vi "Scope_1SDI_v00.vi"(0 "Scope+Safety":T1={"Safety First"={"lim reset"=FALSE, "no limit"=FALSE, "pos slew rate * dt"=12, "neg slew rate * dt"=-12, "Count(Ticks)"=0}, "Scope IPs"={"Trigger Direction"=enum."minus-plus", "Trigger Delay (ms)"=0.0, "Aquisition Rate (kHz)"=4000.0, "Trigger Offset (V)"=0.0, "Scale Offset"={"Scaling"={"Error signal"=1, "Output"=0, "DC Monitor"=1, "Threshold"=1}, "Offset"={"Error Signal"=0, "Output"=0, "DC Monitor"=0, "Threshold"=0}}}}, 9 "Scope":T2, 11 "Lock Select":T4, 13 "XY HD ON":bool, 14 "1SDI Data":u64[](array[numeric])) -> (1 "xy HD A":cluster{i16[], i16[]}(graph), 2 "xy HD B":cluster{i16[], i16[]}(graph), 3 "Scope OP 1SDI":cluster{dbl[], dbl[]}[](graph), 6 "Scope 1SDI ON":bool, 8 "error":dbl[](array[numeric]), 15 "Scope 1SDI FPGA":T3)   [LabVIEW 2013]
doc: "Creates an oscilliscope graph from the FIFO data, as well as packages data structures for FPGA_Cavities via the reference."
uses:
  Strict Type Defs/Lock Select 1SDI.ctl
  Strict Type Defs/Lock or Hold.ctl
  Strict Type Defs/Scope and Safety.ctl
panel:
  out "Scope OPs (for saving)":cluster{dbl[], i16[], i16[], i16[], i16[]}
  in  "Scope":T3={"Trigger Direction"=enum."minus-plus", "Delay"=0, "Aquisition Rate (Ticks)"=20, "Offset"=0, "Channel"=0, "Channel Selector"={"Channel 1"=0, "Channel 2"=0, "Channel 3"=0, "Channel 4"=0}}
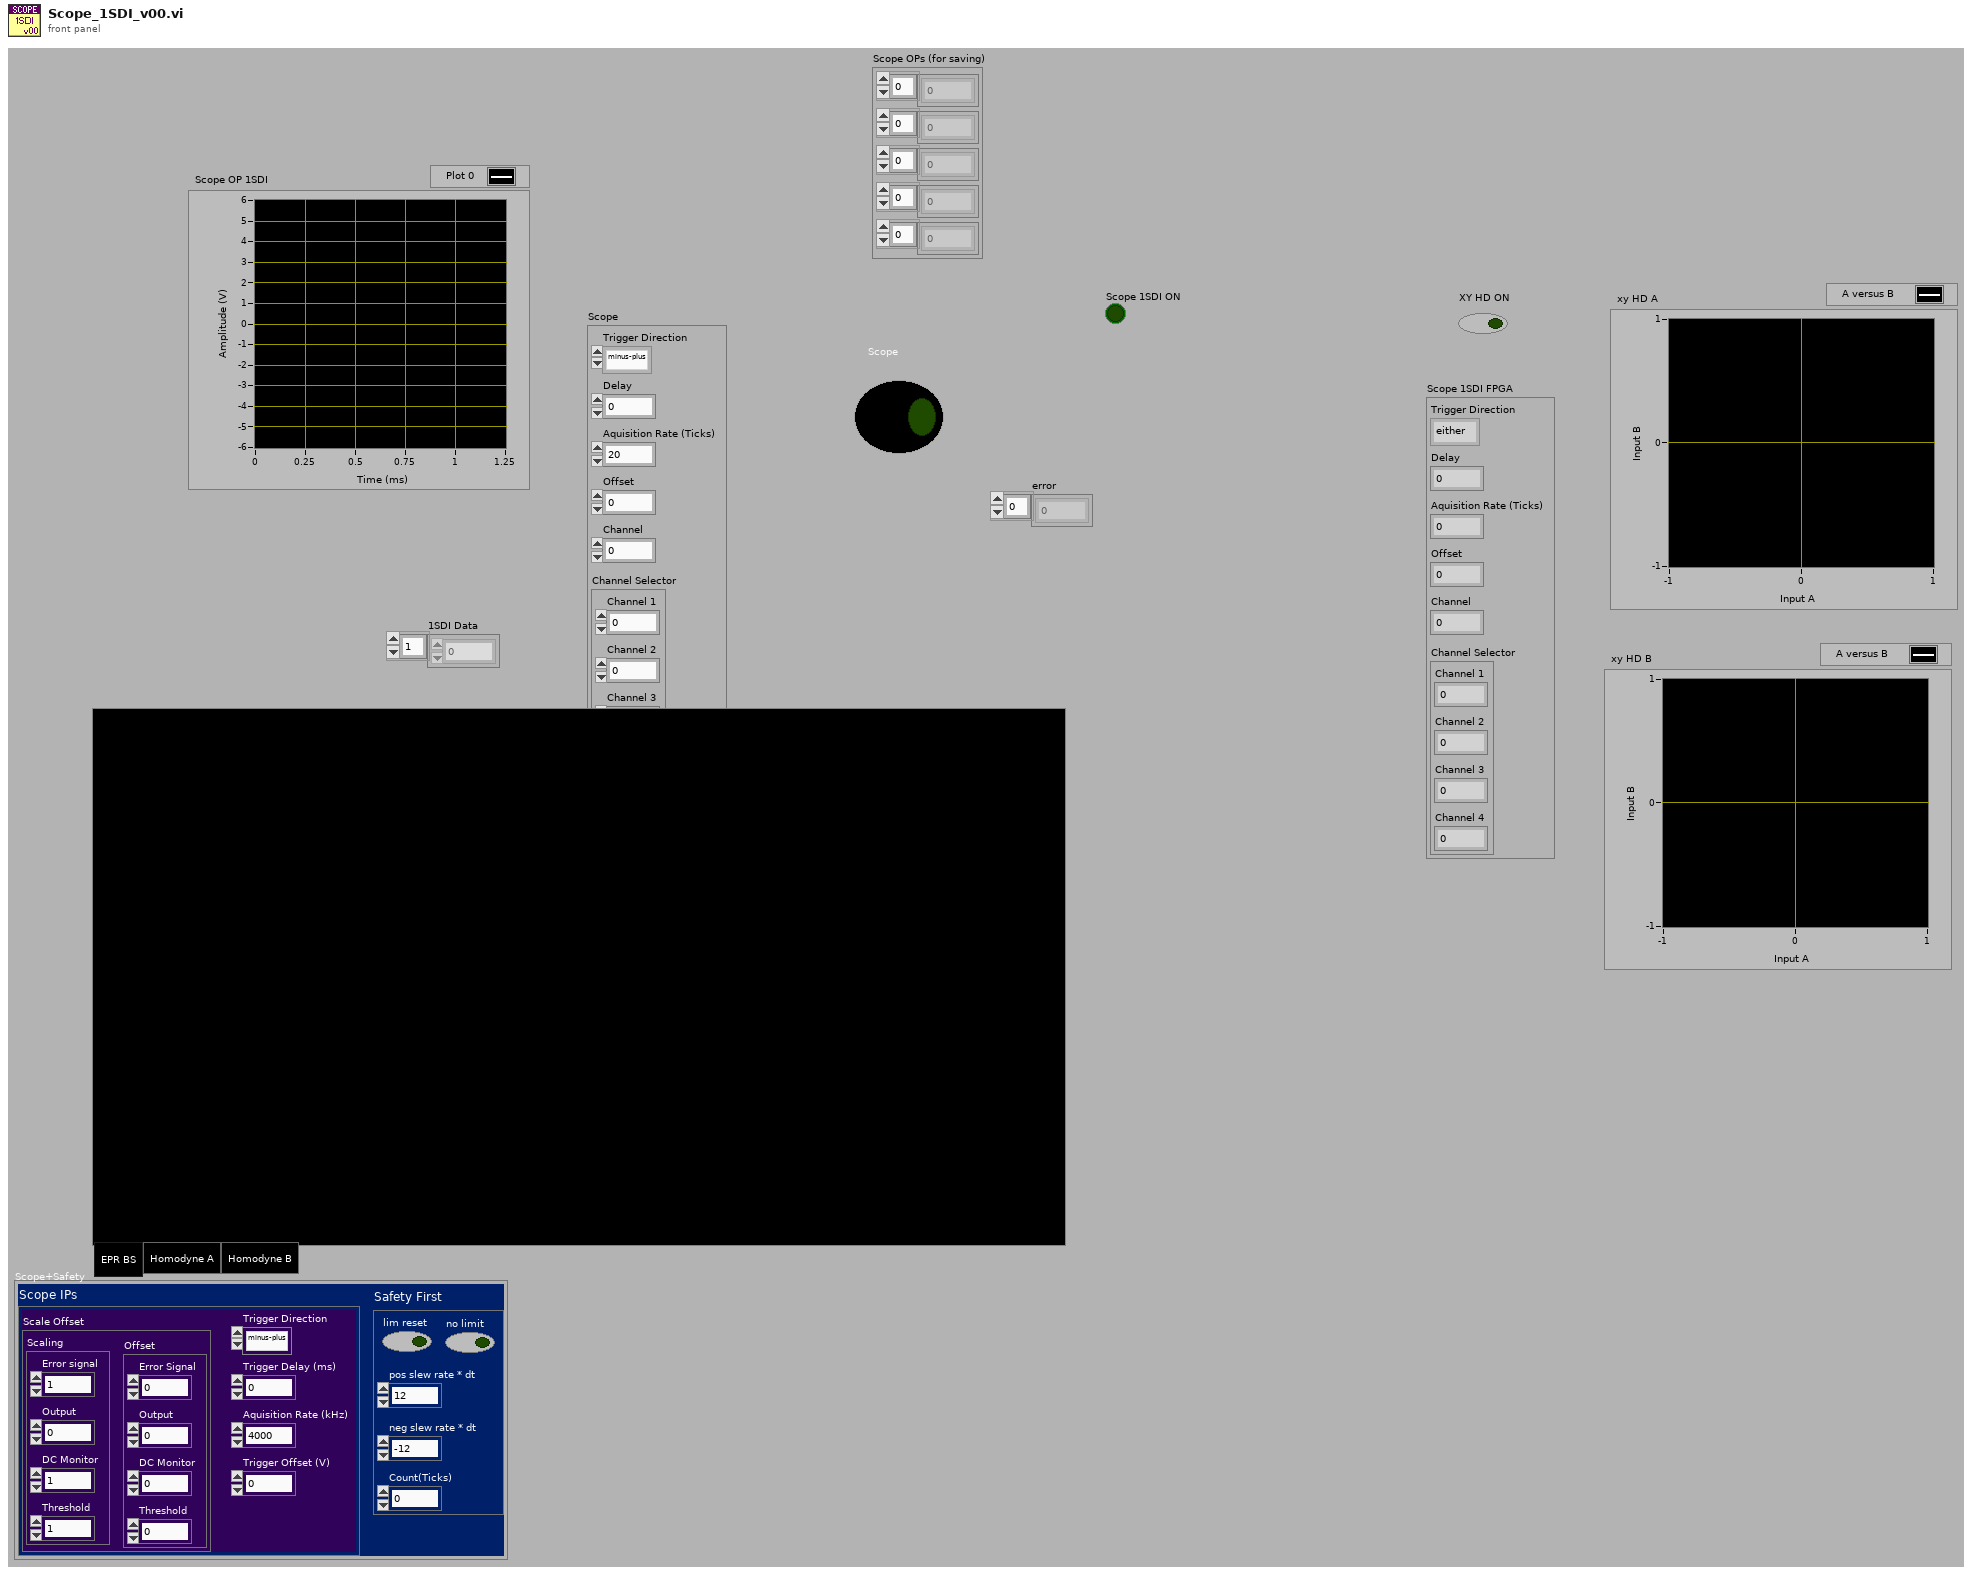
[diagram p1: front panel]
types:
  T1 = typedef "Scope and Safety.ctl" = cluster{"Safety First":cluster{"lim reset":bool, "no limit":bool, "pos slew rate * dt":i16, "neg slew rate * dt":i16, "Count(Ticks)":u32}, "Scope IPs":cluster{"Trigger Direction":enum8{"either", "minus-plus", "plus-minus"}, "Trigger Delay (ms)":dbl, "Aquisition Rate (kHz)":dbl, "Trigger Offset (V)":dbl, "Scale Offset":cluster{"Scaling":cluster{"Error signal":i16, "Output":i16, "DC Monitor":i16, "Threshold":i16}, "Offset":cluster{"Error Signal":i16, "Output":i16, "DC Monitor":i16, "Threshold":i16}}}}
  T2 = typedef "Lock or Hold.ctl" = bool
  T3 = cluster{"Trigger Direction":enum8{"either", "minus-plus", "plus-minus"}, "Delay":u32, "Aquisition Rate (Ticks)":u32, "Offset":i16, "Channel":i32, "Channel Selector":cluster{"Channel 1":i32, "Channel 2":i32, "Channel 3":i32, "Channel 4":i32}}
  T4 = typedef "Lock Select 1SDI.ctl" = enum32{"EPR BS", "Homodyne A", "Homodyne B"}
  T5 = cluster{"Channel 1":i32, "Channel 2":i32, "Channel 3":i32, "Channel 4":i32}
  T6 = cluster{"Trigger Direction":enum8{"either", "minus-plus", "plus-minus"}, "Trigger Delay (ms)":dbl, "Aquisition Rate (kHz)":dbl, "Trigger Offset (V)":dbl, "Scale Offset":cluster{"Scaling":cluster{"Error signal":i16, "Output":i16, "DC Monitor":i16, "Threshold":i16}, "Offset":cluster{"Error Signal":i16, "Output":i16, "DC Monitor":i16, "Threshold":i16}}}
  T7 = cluster{"Error signal":i16, "Output":i16, "DC Monitor":i16, "Threshold":i16}
  T8 = cluster{"Error Signal":i16, "Output":i16, "DC Monitor":i16, "Threshold":i16}
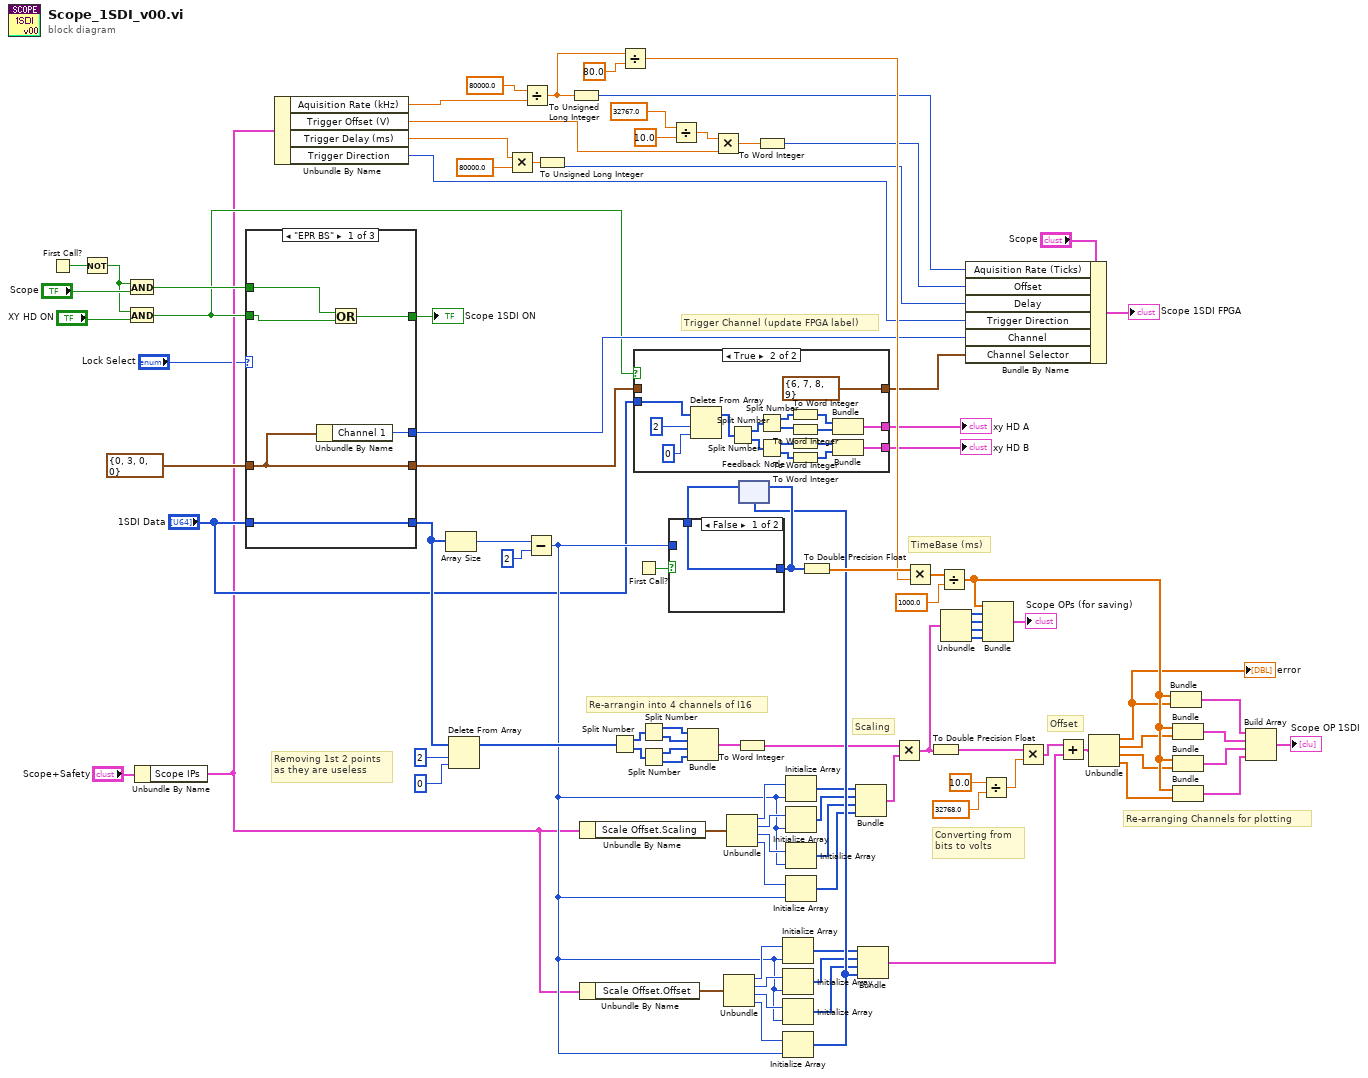
[diagram p0: block diagram]
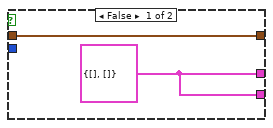
[diagram p2: hidden frame]
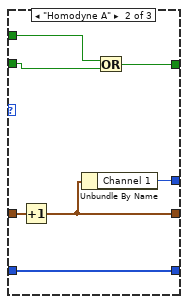
[diagram p4: hidden frame]
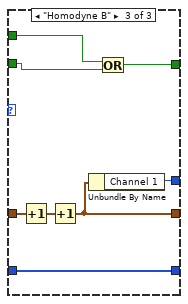
[diagram p5: hidden frame]
diagram:
  # "Trigger Channel (update FPGA label)"
  # "TimeBase (ms)"
  # "Re-arranging Channels for plotting"
  # "Re-arrangin into 4 channels of I16"
  # "Converting from\nbits to volts"
  # "Offset"
  # "Scaling"
  # "Removing 1st 2 points\nas they are useless"
  n1 = First Call?() -> (First Call?: T/F=w17:bool)
  n2 = Not(x=w17) -> (.not. x?=w11:bool)
  n3 = And(x=w11, y="Scope") -> (x .and. y?=w16:T2)
  n4 = And(x=w11, y="XY HD ON") -> (x .and. y?=w8:bool)
  n5 = Unbundle By Name("Scope+Safety") -> ("Scope IPs"=w3:T6)
  n6 = case shown="\"EPR BS\"" "Lock Select" {
    tunnel: [w105 w111 w115] -> w26
    tunnel: "1SDI Data" -> [w105 w111 w115]
    tunnel: [w100 w107 w114] -> w19
    tunnel: T5 {"Channel 1"=0, "Channel 2"=3, "Channel 3"=0, "Channel 4"=0} ("Channel Selector") -> [w101 w112 w120]
    tunnel: [w101 w106 w113] -> w10
    tunnel: w16 -> [w102 w108 w116]
    tunnel: [w104 w110 w118] -> w14
    tunnel: w8 -> [w103 w109 w117]
    frame "EPR BS" {
      n7 = Unbundle By Name(w101) -> ("Channel 1"=w100:i32)
      n8 = Or(x=w102, y=w103) -> (x .or. y?=w104:T2)
    }
    frame "Homodyne A" {
      n9 = Increment(x=w112) -> (x+1=w106:T5)
      n10 = Unbundle By Name(w106) -> ("Channel 1"=w107:i32)
      n11 = Or(x=w108, y=w109) -> (x .or. y?=w110:T2)
    }
    frame "Homodyne B" {
      n12 = Increment(x=w120) -> (x+1=w119:T5)
      n13 = Increment(x=w119) -> (x+1=w113:T5)
      n14 = Unbundle By Name(w113) -> ("Channel 1"=w114:i32)
      n15 = Or(x=w116, y=w117) -> (x .or. y?=w118:T2)
    }
  }
  "Scope 1SDI ON" <- w14
  n16 = Unbundle By Name(w3) -> ("Aquisition Rate (kHz)"=w98:dbl, "Trigger Offset (V)"=w93:dbl, "Trigger Delay (ms)"=w91:dbl, "Trigger Direction"=w20:enum8{"either", "minus-plus", "plus-minus"})
  n17 = Array Size(array=w26) -> (size(s)=w84:i32)
  n18 = Delete From Array(array=w26, length=2, index=0) -> (array with subset deleted=w30:u64[])  [unwired: 1 out]
  n19 = Multiply(x=w91, y=80000.0) -> (x*y=w92:dbl)
  n20 = Divide(x=80000.0, y=w98) -> (x/y=w88:dbl)
  n21 = Subtract(x=w84, y=2) -> (x-y=w13:i32)
  n22 = To Unsigned Long Integer(number=w92) -> (unsigned 32bit integer=w21:u32)
  n23 = To Unsigned Long Integer(number=w88) -> (unsigned 32bit integer=w23:u32)
  n24 = Unbundle By Name(w3) -> ("Scale Offset.Scaling"=w55:T7)
  n25 = Unbundle By Name(w3) -> ("Scale Offset.Offset"=w39:T8)
  n26 = Split Number(x=w30) -> (hi(x)=w32:u32[], lo(x)=w31:u32[])
  n27 = Divide(x=w88, y=80.0) -> (x/y=w29:dbl)
  n28 = case shown="True" w8 {
    tunnel: w10 -> [w122 _]
    tunnel: [w122 T5 {"Channel 1"=6, "Channel 2"=7, "Channel 3"=8, "Channel 4"=9} ("Channel Selector")] -> w9
    tunnel: "1SDI Data" -> [_ w124]
    tunnel: [w121 w128] -> w7
    tunnel: [w121 w127] -> w6
    frame False {
      w121 = cluster{i16[], i16[]} {[], []}
    }
    frame True {
      n29 = Delete From Array(array=w124, length=2, index=0) -> (array with subset deleted=w123:u64[])  [unwired: 1 out]
      n30 = Split Number(x=w123) -> (hi(x)=w137:u32[], lo(x)=w133:u32[])
      n31 = Split Number(x=w137) -> (hi(x)=w138:u16[], lo(x)=w136:u16[])
      n32 = Split Number(x=w133) -> (hi(x)=w132:u16[], lo(x)=w131:u16[])
      n33 = To Word Integer(number=w138) -> (16bit integer=w135:i16[])
      n34 = To Word Integer(number=w136) -> (16bit integer=w134:i16[])
      n35 = To Word Integer(number=w132) -> (16bit integer=w129:i16[])
      n36 = To Word Integer(number=w131) -> (16bit integer=w130:i16[])
      n37 = Bundle(w135, w134) -> (w128:cluster{i16[], i16[]})  [unwired: 1 in]
      n38 = Bundle(w129, w130) -> (w127:cluster{i16[], i16[]})  [unwired: 1 in]
    }
  }
  "xy HD A" <- w7
  "xy HD B" <- w6
  n39 = First Call?() -> (First Call?: T/F=w58:bool)
  n40 = Split Number(x=w32) -> (hi(x)=w80:u16[], lo(x)=w81:u16[])
  n41 = Split Number(x=w31) -> (hi(x)=w82:u16[], lo(x)=w83:u16[])
  n42 = Divide(x=32767.0, y=10.0) -> (x/y=w96:dbl)
  n43 = Bundle(w80, w81, w82, w83) -> (w56:cluster{u16[], u16[], u16[], u16[]})  [unwired: 1 out]
  n44 = Multiply(x=w96, y=w93) -> (x*y=w97:dbl)
  n45 = Unbundle(w39) -> ("Error Signal"=w38:i16, "Output"=w42:i16, "DC Monitor"=w41:i16, "Threshold"=w40:i16)
  n46 = Unbundle(w55) -> ("Error signal"=w52:i16, "Output"=w51:i16, "DC Monitor"=w53:i16, "Threshold"=w54:i16)
  n47 = To Word Integer(number=w56) -> (16bit integer=w57:cluster{i16[], i16[], i16[], i16[]})
  n48 = To Word Integer(number=w97) -> (16bit integer=w22:i16)
  n49 = Initialize Array(w38, w13) -> (w43:i16[])
  n50 = Initialize Array(w42, w13) -> (w44:i16[])
  n51 = Initialize Array(w41, w13) -> (w45:i16[])
  n52 = Initialize Array(w40, w13) -> (w59:i16[])
  n53 = feedback #1(w59) -> (w60:i32[])
  n54 = case shown="False" w58 {
    tunnel: w13 -> [_ w142]
    tunnel: [w140 w141] -> w61
    tunnel: w60 -> [w140 _]
    frame False {
    }
    frame True {
      n55 = for {
        N: w142 -> [_]
        tunnel: [w143] -> w141 mode=indexing
        i -> [w143]
      }
    }
  }
  n56 = feedback-in #1(w61) -> ()
  n57 = Initialize Array(w52, w13) -> (w50:i16[])
  n58 = Initialize Array(w51, w13) -> (w49:i16[])
  n59 = Initialize Array(w53, w13) -> (w48:i16[])
  n60 = Initialize Array(w54, w13) -> (w47:i16[])
  n61 = To Double Precision Float(number=w61) -> (double precision float=w62:dbl[])
  n62 = Bundle(w50, w49, w48, w47) -> (w46:cluster{i16[], i16[], i16[], i16[]})  [unwired: 1 out]
  n63 = Bundle(w43, w44, w45, w59) -> (w37:cluster{i16[], i16[], i16[], i16[]})  [unwired: 1 out]
  n64 = Multiply(x=w57, y=w46) -> (x*y=w73:cluster{i16[], i16[], i16[], i16[]})
  n65 = Multiply(x=w62, y=w29) -> (x*y=w63:dbl[])
  n66 = To Double Precision Float(number=w73) -> (double precision float=w28:cluster{dbl[], dbl[], dbl[], dbl[]})
  n67 = Divide(x=w63, y=1000.0) -> (x/y=w78:dbl[])
  n68 = Unbundle(w73) -> (w74:i16[], w75:i16[], w76:i16[], w77:i16[])
  n69 = Bundle By Name(cluster="Scope", "Aquisition Rate (Ticks)"=w23, "Offset"=w22, "Delay"=w21, "Trigger Direction"=w20, "Channel"=w19, "Channel Selector"=w9) -> (→"Scope 1SDI FPGA":T3)
  n70 = Divide(x=10.0, y=32768.0) -> (x/y=w27:dbl)
  n71 = Bundle(w78, w74, w75, w76, w77) -> (→"Scope OPs (for saving)":cluster{dbl[], i16[], i16[], i16[], i16[]})  [unwired: 1 in]
  n72 = Multiply(x=w28, y=w27) -> (x*y=w35:cluster{dbl[], dbl[], dbl[], dbl[]})
  n73 = Add(x=w35, y=w37) -> (x+y=w36:cluster{dbl[], dbl[], dbl[], dbl[]})
  n74 = Unbundle(w36) -> (w1:dbl[], w65:dbl[], w66:dbl[], w67:dbl[])
  "error" <- w1
  n75 = Bundle(w78, w1) -> (w68:cluster{dbl[], dbl[]})  [unwired: 1 in]
  n76 = Bundle(w78, w65) -> (w69:cluster{dbl[], dbl[]})  [unwired: 1 in]
  n77 = Bundle(w78, w66) -> (w70:cluster{dbl[], dbl[]})  [unwired: 1 in]
  n78 = Bundle(w78, w67) -> (w71:cluster{dbl[], dbl[]})  [unwired: 1 in]
  n79 = Build Array(w68, w69, w70, w71) -> (→"Scope OP 1SDI":cluster{dbl[], dbl[]}[])
